vi "SB -Set - get DIO port A, B, C bit status.vi"(1 "Configure DIO\nports - set":dbl format="%.2f", 3 "error in":errorcluster, 4 "Action":bool, 5 "Address / Port":i16=1 min=1 max=31 step=1) -> (0 "error out":errorcluster, 2 "Report current DIO port\nsetting - read":string)   [LabVIEW 2014]
panel:
  # "Read"
  # "Write"
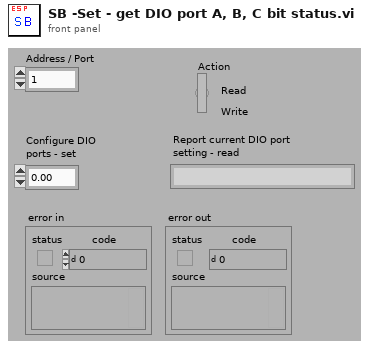
[diagram p1: front panel]
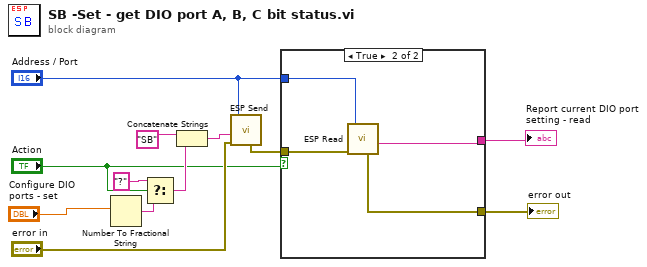
[diagram p0: block diagram]
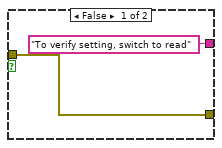
[diagram p2: hidden frame]
diagram:
  n1 = Number To Fractional String(number="Configure DIO\nports - set") -> (F-format string=w9:string)  [unwired: 3 in]
  n2 = Select(t="?", s="Action", f=w9) -> (s? t:f=w10:string)
  n3 = Concatenate Strings("SB" ("Substring"), w10) -> (w11:string)
  n4 = call "ESP Send.vi"("Address / Port"="Address / Port", "Command String"=w11, "error in"="error in") -> ("error out"=w4:errorcluster)  [unwired: 5 in]
  n5 = case shown="True" "Action" {
    tunnel: "Address / Port" -> [_ w18]
    tunnel: w4 -> [w14 w17]
    tunnel: [w14 w16] -> w3
    tunnel: ["To verify setting, switch to read" w15] -> w1
    frame False {
    }
    frame True {
      n6 = call "ESP Read.vi"("Address / Port"=w18, "error in"=w17) -> ("error out"=w16:errorcluster, "Response String"=w15:string)  [unwired: 5 in]
    }
  }
  "error out" <- w3
  "Report current DIO port\nsetting - read" <- w1
